vi "charts and graphs and loops.vi"() -> ()   [LabVIEW 2014]
panel:
  out "Waveform Graph":dbl[](graph)
  in  "?":bool
  out "Temperature Value (C)":dbl
  out "Waveform Chart":dbl(graph)
  in  "Tmeperature (F)":dbl(slide) scale=0.0..200.0
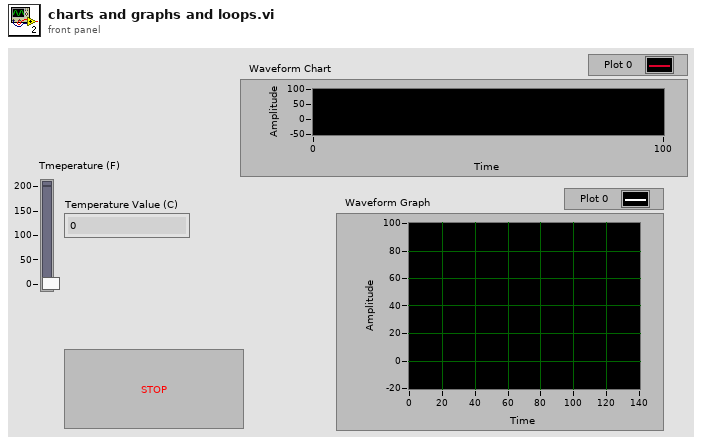
[diagram p1: front panel]
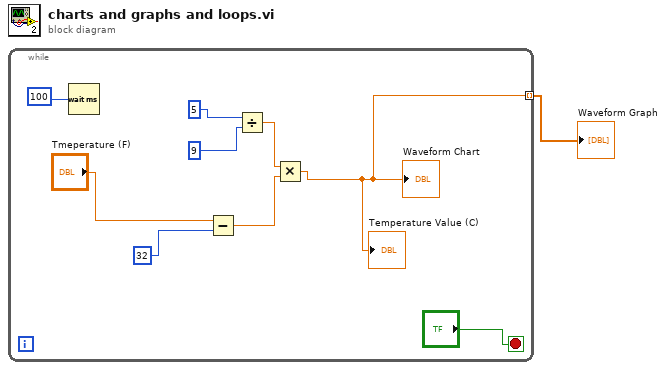
[diagram p0: block diagram]
diagram:
  n1 = while {
    tunnel: [w2] -> w1 mode=indexing
    stop <- "?" stop-if-true
    n2 = Wait (ms)(milliseconds to wait=100) -> ()  [unwired: 1 out]
    n3 = Subtract(x="Tmeperature (F)", y=32) -> (x-y=w7:dbl)
    n4 = Divide(x=5, y=9) -> (x/y=w4:dbl)
    n5 = Multiply(x=w4, y=w7) -> (x*y=w2:dbl)
    "Waveform Chart" <- w2
    "Temperature Value (C)" <- w2
  }
  "Waveform Graph" <- w1
